vi "Spartan Client Version.vi"() -> ()   [LabVIEW 2011]
uses:
  SI.LIB/OGAB Version.ctl
panel:
  in  "Data Path":path
  in  "ServerPort":u16=80
  out "STOP":bool
  in  "Test Timeout (ms)":i32=1800000
  in  "SERVER":string
  in  "Version":T1={"Version"="6.3", "Build Number"=12, "Build Date/Time"=3440694548.419435} {"Build Date/Time" format="%<%X\n%x>T"}
  # "Note: The version\nglobal is set during\nbuild.  Don't change\nor rename this variable"
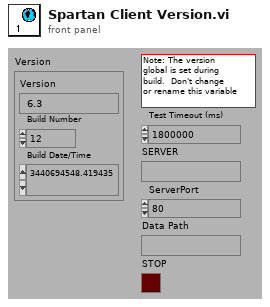
[diagram p1: front panel]
types:
  T1 = typedef "OGAB Version.ctl" = cluster{"Version":string, "Build Number":u32, "Build Date/Time":dbl}
diagram:
